vi "LTESaveDataReal2.vi"(7 "Boolean":bool, 8 "error in":errorcluster, 9 "varName":string, 10 "real2":dbl[][](array[numeric]), 11 "Path":path=path "C:/Users/Administrator/Desktop") -> (0 "error IO":errorcluster)   [LabVIEW 2015]
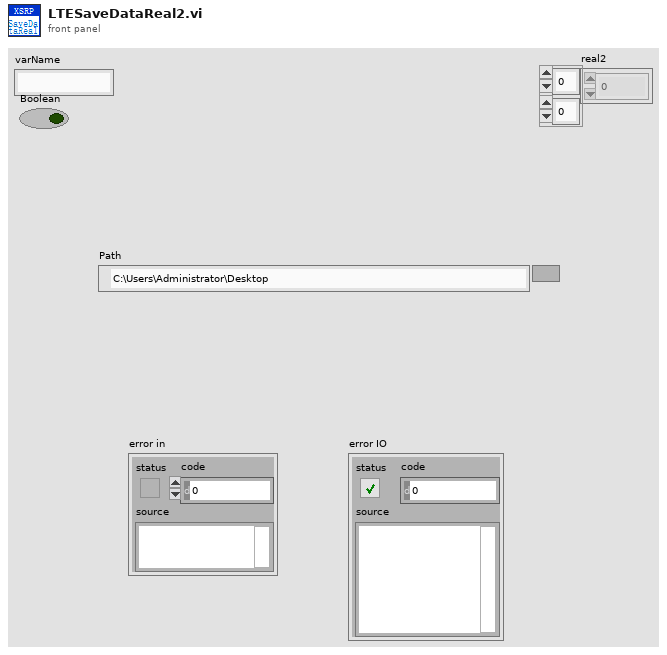
[diagram p1: front panel]
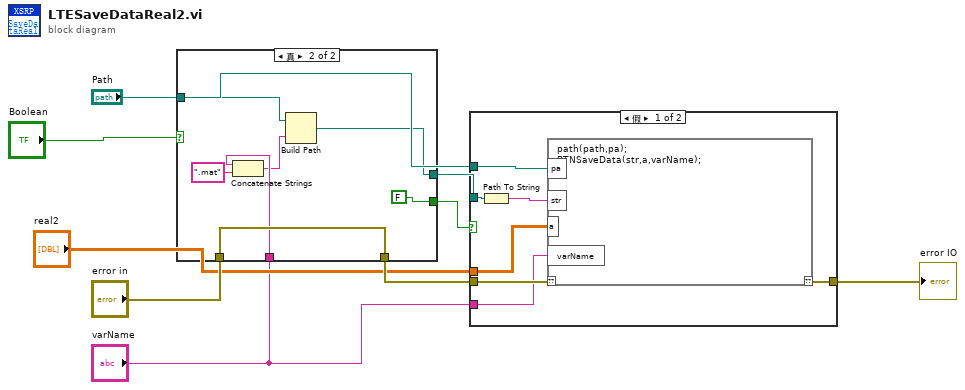
[diagram p0: block diagram]
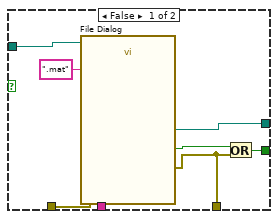
[diagram p2: hidden frame]
diagram:
  n1 = case shown="真" "Boolean" {
    tunnel: [w16 w20] -> w9
    tunnel: [w14 FALSE] -> w8
    tunnel: "Path" -> [w13 w21]
    tunnel: "error in" -> [w12 w23]
    tunnel: [w11 w23] -> w4
    tunnel: "varName" -> [_ w18]
    frame False {
      n2 = call "File Dialog"("start path"=w13, "error in"=w12, "pattern (all files)"=".mat") -> ("selected path"=w16:path, "cancelled"=w10:bool, "error out"=w11:errorcluster)  [unwired: 9 in, 1 out]
      n3 = Or(x=w10, y=w11) -> (x .or. y?=w14:bool)
    }
    frame True {
      n4 = Concatenate Strings(w18, ".mat" ("string")) -> (w17:string)
      n5 = Build Path(base path=w21, name or relative path=w17) -> (appended path=w20:path)
    }
  }
  n6 = case shown="假" w8 {
    tunnel: w9 -> [w30 _]
    tunnel: "Path" -> [w28 _]
    tunnel: w4 -> [w27 w31]
    tunnel: [w26 w31] -> w6
    tunnel: "real2" -> [w25 _]
    tunnel: "varName" -> [w24 _]
    frame False {
      n7 = Path To String(path=w30) -> (string=w29:string)
      n8 = script code="path(path,pa);\nBTNSaveData(str,a,varName);"("??"=w27, "pa"=w28, "a"=w25, "str"=w29, "varName"=w24) -> ("??"=w26:errorcluster)
    }
    frame True {
    }
  }
  "error IO" <- w6
